vi "Read PreparePassPlaysEnum.vi"(8 "error in (no error)":errorcluster, 11 "Ally in":refnum<class "Ally.lvclass">) -> (0 "error out":errorcluster, 2 "PreparePassPlaysEnum":T1[](array[typedef])=[enum."PreparePass", enum."PrepareDoublePass"], 3 "Ally out":refnum<class "Ally.lvclass">)   [LabVIEW 2020, in "Ally.lvclass"]
uses:
  Ally.lvclass
  Team_class/OffensivePlay.ctl
  Ally.lvclass/Ally.ctl
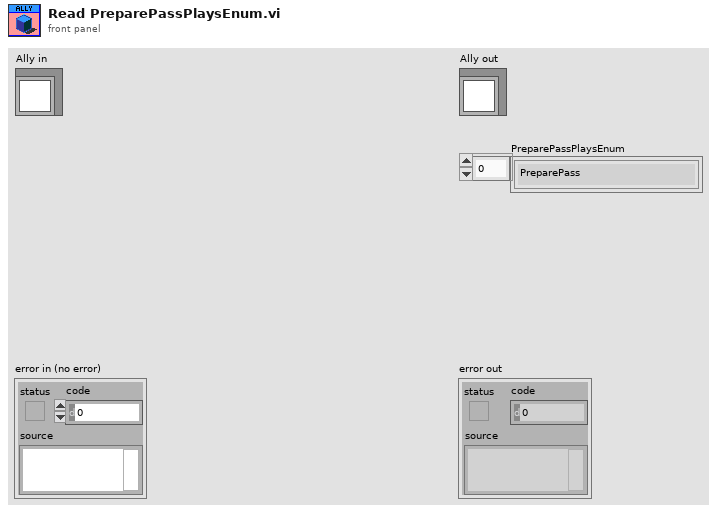
[diagram p1: front panel]
types:
  T1 = typedef "OffensivePlay.ctl" = enum16{"PrepareFourthPass", "KeeperPassToStriker", "PrepareKeeperPass", "ACBPass", "ABCPass", "PrepareTriplePass", "TableWithStriker", "TableWith2ndStrikerPlay", "PrepareDoublePass", "PrepareRollToPass", "SimplePass", "PreparePass", "PassToStriker", "BallOutOfField", "PassTo2ndStriker", "StopOffensive", "Prepare Penalty Enemy", "EnemyPossessionAtEnemyField", "EnemyPossesionAtOurField", "TestPlay", "PreparePenaltyAlly", "KickPenaltyAlly", "PrepareKickoffAlly", "PrepareKickoffEnemy", "IndirectEnemy", "DirectEnemy", "PreparePassInGame1", "NormalGame", "DirectKick", "Pass", "Halt", "Timeout", "PassPlay", "PenaltyEnemy"}
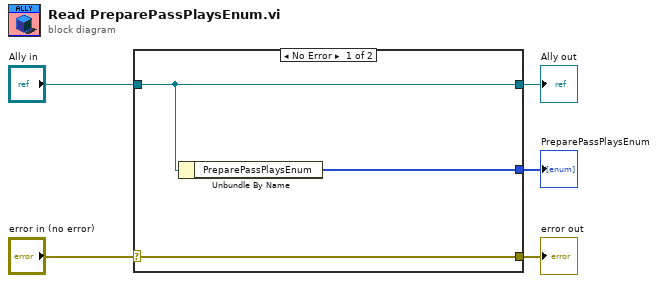
[diagram p0: block diagram]
diagram:
  n1 = case shown="No Error" "error in (no error)" {
    selector: "error in (no error)" -> [w8 w9]
    tunnel: [w8 w9] -> w4
    tunnel: [w7 w10] -> w2
    tunnel: "Ally in" -> [w7 w10]
    tunnel: [w6 _] -> w1
    frame No Error {
      n2 = Unbundle By Name(w7) -> ("PreparePassPlaysEnum"=w6:T1[])
    }
    frame Error {
    }
  }
  "error out" <- w4
  "Ally out" <- w2
  "PreparePassPlaysEnum" <- w1
